vi "GetURI&Port.vi"(0 "URI in":string) -> (1 "Port":u16, 2 "URI":string)   [LabVIEW 2012]
doc: "Returns the URI port"
uses:
  <vilib>/regexp/Match Regular Expression.xnode
  _ROSDefinition.vi
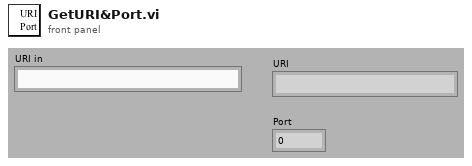
[diagram p1: front panel]
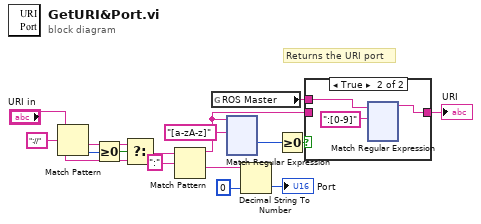
[diagram p0: block diagram]
diagram:
  # "Returns the URI port"
  n1 = Match Pattern(string="URI in", regular expression="://") -> (after substring=w9:string, offset past match=w11:i32)  [unwired: 1 in, 2 out]
  n2 = Greater Or Equal To 0?(x=w11) -> (x >= 0?=w10:bool)
  n3 = Select(t=w9, s=w10, f="URI in") -> (s? t:f=w7:string)
  n4 = Match Pattern(string=w7, regular expression=":") -> (before substring=w3:string, after substring=w14:string)  [unwired: 1 in, 2 out]
  n5 = global read "_ROSDefinition.vi" "ROS Master"() -> (w1:string)
  n6 = xnode "Match Regular Expression"("input string"=w3, "regular expression"="[a-zA-z]") -> ("offset past match"=w5:i32)  [unwired: 4 in, 4 out]
  n7 = Decimal String To Number(string=w14, default (0L)=u16 0 ("default (0 I32)")) -> (number=→"Port":u16)  [unwired: 1 in, 1 out]
  n8 = Greater Or Equal To 0?(x=w5) -> (x >= 0?=w4:bool)
  n9 = case shown="True" w4 {
    tunnel: w3 -> [w17 _]
    tunnel: [w17 w18] -> w2
    tunnel: w1 -> [_ w20]
    frame False {
    }
    frame True {
      n10 = xnode "Match Regular Expression"("input string"=w20, "regular expression"=":[0-9]") -> ("before match"=w18:string)  [unwired: 4 in, 4 out]
    }
  }
  "URI" <- w2
